vi "ParseTree_Add_Child.vi"(8 "index of child":i32, 9 "child":i32, 10 "parent":u32, 11 "Parse Tree in":T1[](array[typedef])) -> (3 "Parse Tree out":T1[](array[typedef]))   [LabVIEW 2021]
uses:
  <resource>/MathScriptParser/Statement.ctl
  <resource>/MathScriptParser/NodeType.ctl
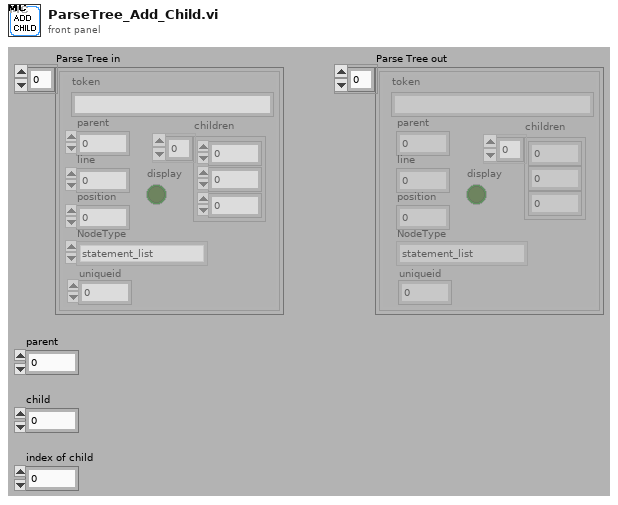
[diagram p1: front panel]
types:
  T1 = typedef "Statement.ctl" = cluster{"parent":u32, "children":u32[], "token":string, "NodeType":T2, "line":u32, "display":bool, "position":u32, "uniqueid":u32}
  T2 = typedef "NodeType.ctl" = enum16{"statement_list", "expression_list", "matrix", "row", "command", "function_1_1", "function_1_N", "function_N_1", "function_N_N", "operator", "assignment", "for", "if", "switch", "while", "try", "range", "identifier", "struct_field", "constant", "udfunction_1_1", "udfunction_1_N", "udfunction_N_1", "udfunction_N_N", "udfunction_0_0", "udfunction_0_1", "udfunction_0_N", "udfunction_1_0", "udfunction_N_0", "function_0_1", "function_0_N", "struct_ref", "array_ref", "cell_array_ref", "cell_matrix"}
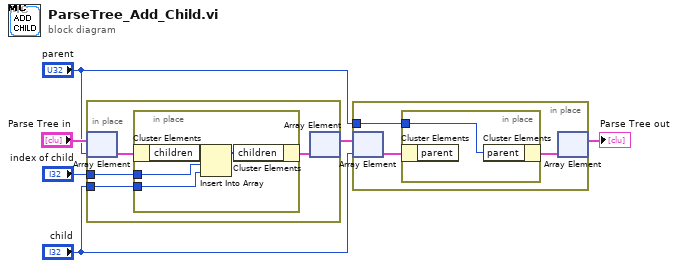
[diagram p0: block diagram]
diagram:
  n1 = in-place {
    in-place-border: "child" -> [w10]
    in-place-border: "index of child" -> [w9]
    n2 = in-place-array #1("Parse Tree in", "parent") -> (w8:T1)
    n3 = in-place {
      in-place-border: w10 -> [w11]
      in-place-border: w9 -> [w12]
      n4 = in-place-cluster #2(w8) -> ("children"=w14:u32[])
      n5 = Insert Into Array(array=w14, index=w12, new element=w11) -> (w13:u32[])
      n6 = in-place-cluster #2("children"=w13) -> (w7:T1)
    }
    n7 = in-place-array #1(w7) -> (w4:T1[])  [unwired: 1 out]
  }
  n8 = in-place {
    in-place-border: "parent" -> [w17]
    n9 = in-place-array #3(w4, "child") -> (w16:T1)
    n10 = in-place {
      in-place-border: w17 -> [w18]
      n11 = in-place-cluster #4(w16) -> ()  [unwired: 1 out]
      n12 = in-place-cluster #4("parent"=w18) -> (w15:T1)
    }
    n13 = in-place-array #3(w15) -> (→"Parse Tree out":T1[])  [unwired: 1 out]
  }
